vi "PID Initializer.vi"(8 "error in":errorcluster, 10 "PIDF":cluster{"P":dbl, "I":dbl, "D":dbl, "F":dbl} {"F" format="%#_13g"; "D" format="%#_13g"; "I" format="%#_13g"; "P" format="%#_13g"}, 11 "Can IDs":T7) -> (0 "error out":errorcluster, 3 "Motors":T6)   [LabVIEW 2020]
uses:
  <vilib>/Rock Robotics/WPI/MotorControl/WPI_MotorControlDeviceRef.ctl
  <vilib>/Rock Robotics/WPI/MotorControl/WPI_MotorControlType.ctl
  <vilib>/Rock Robotics/SystemInterfaces/DIO/FPGA_DIOPWMChannel.ctl
  <vilib>/Rock Robotics/WPI/PWM/WPI_PWMDeadband.ctl
  <vilib>/Rock Robotics/SystemInterfaces/DIO/FPGA_DIOChannel.ctl
  <vilib>/Rock Robotics/WPI/ThirdParty/Phoenix-LabVIEW/Motor Controller/Controls/CTRE_Phoenix_MotorControl_NeutralMode.ctl
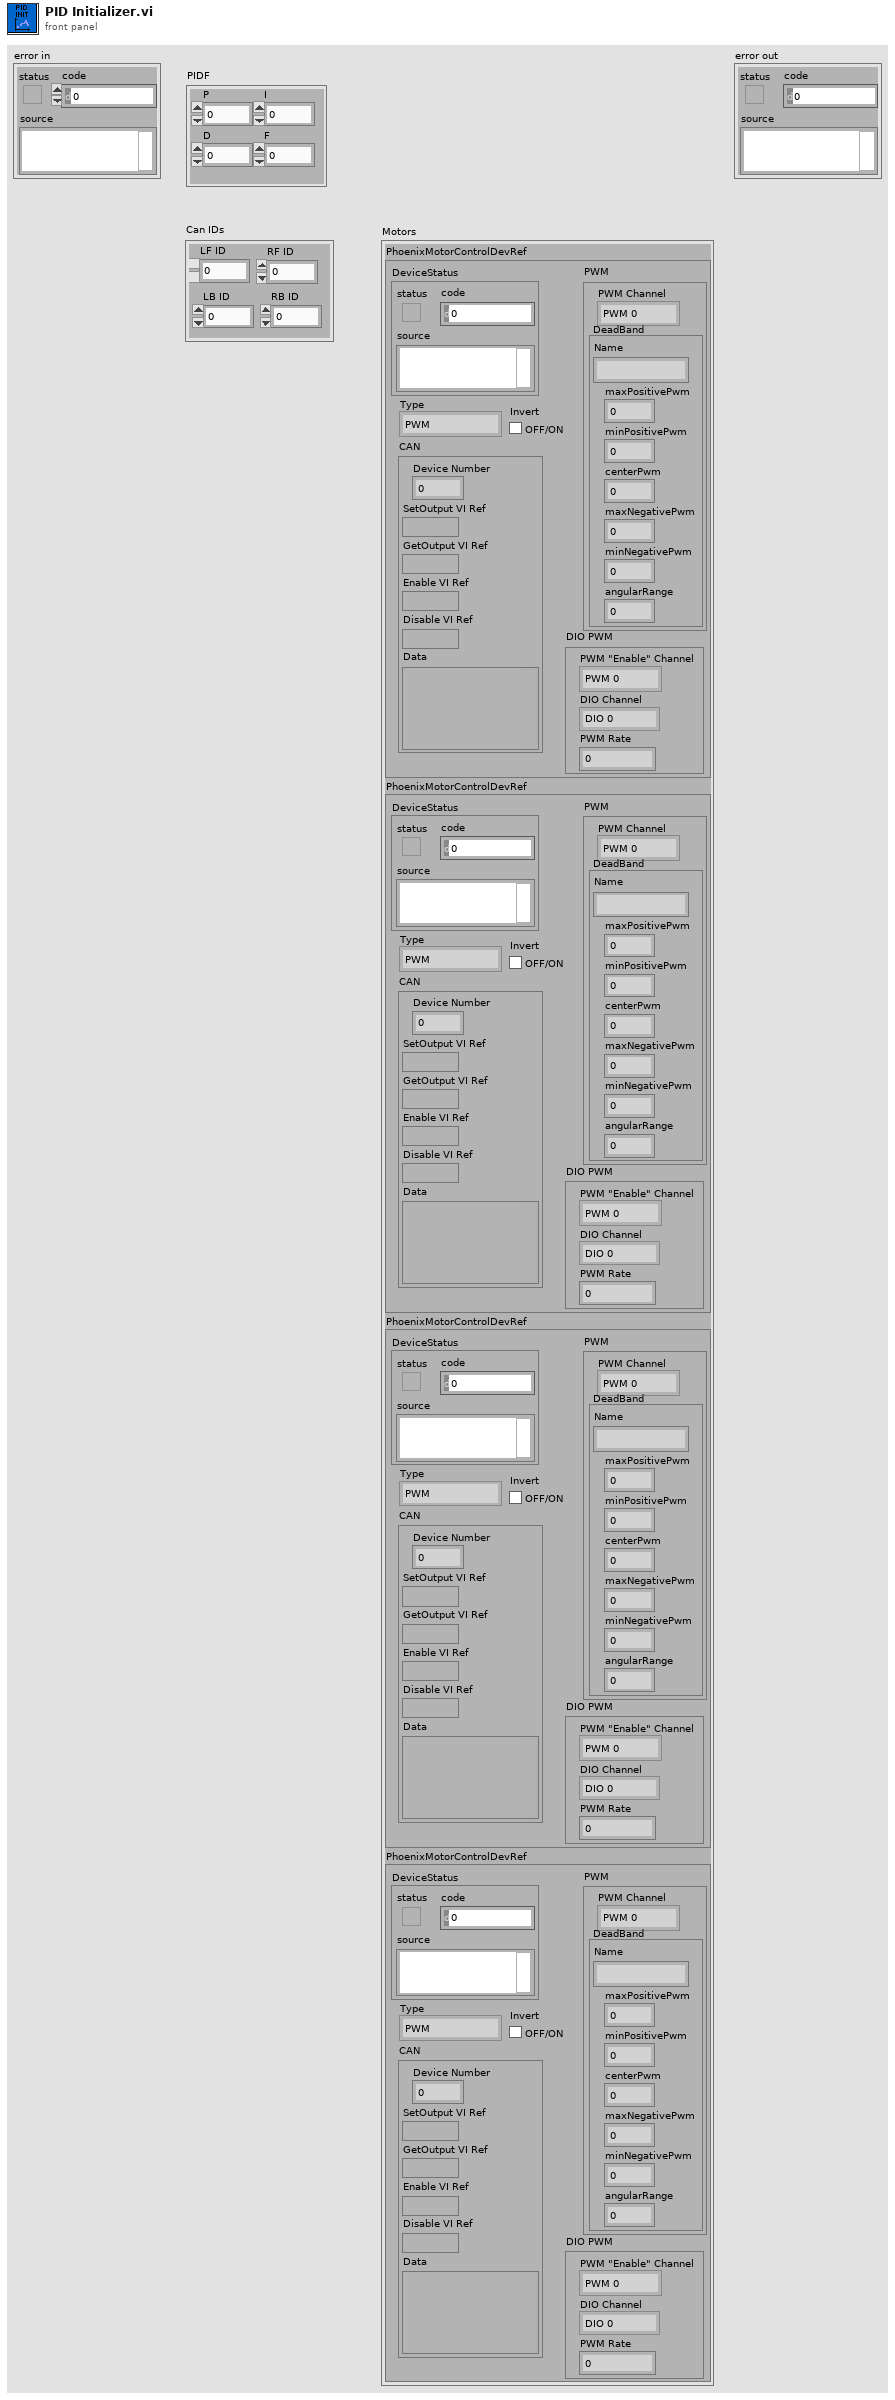
[diagram p1: front panel]
types:
  T1 = typedef "WPI_MotorControlDeviceRef.ctl" = cluster{"DeviceStatus":errorcluster, "Type":T2, "PWM":cluster{"PWM Channel":T3, "DeadBand":T4}, "CAN":cluster{"Device Number":u8, "SetOutput VI Ref":variant, "GetOutput VI Ref":variant, "Enable VI Ref":variant, "Disable VI Ref":variant, "Data":variant}, "Invert":bool, "DIO PWM":cluster{"PWM \"Enable\" Channel":T3, "DIOChannel":T5, "PWM Rate":dbl}}
  T2 = typedef "WPI_MotorControlType.ctl" = enum16{"PWM", "CAN", "DIO PWM"}
  T3 = typedef "FPGA_DIOPWMChannel.ctl" = enum8{"PWM 0", "PWM 1", "PWM 2", "PWM 3", "PWM 4", "PWM 5", "PWM 6", "PWM 7", "PWM 8", "PWM 9", "PWM MXP 0", "PWM MXP 1", "PWM MXP 2", "PWM MXP 3", "PWM MXP 4", "PWM MXP 5", "PWM MXP 6", "PWM MXP 7", "PWM MXP 8", "PWM MXP 9", "Invalid"}
  T4 = typedef "WPI_PWMDeadband.ctl" = cluster{"Name":string, "maxPositivePwm":i32, "minPositivePwm":i32, "centerPwm":i32, "maxNegativePwm":i32, "minNegativePwm":i32, "angularRange":u16}
  T5 = typedef "FPGA_DIOChannel.ctl" = enum8{"DIO 0", "DIO 1", "DIO 2", "DIO 3", "DIO 4", "DIO 5", "DIO 6", "DIO 7", "DIO 8", "DIO 9", "DIO MXP 0", "DIO MXP 1", "DIO MXP 2", "DIO MXP 3", "DIO MXP 4", "DIO MXP 5", "DIO MXP 6", "DIO MXP 7", "DIO MXP 8", "DIO MXP 9", "DIO MXP 10", "DIO MXP 11", "DIO MXP 12", "DIO MXP 13", "DIO MXP 14", "DIO MXP 15", "SPI Port CS1", "SPI Port CS2", "SPI Port CS3", "SPI Port MISO", "SPI Port MOSI", "Invalid"}
  T6 = cluster{"PhoenixMotorControlDevRef":T1, "PhoenixMotorControlDevRef":T1, "PhoenixMotorControlDevRef":T1, "PhoenixMotorControlDevRef":T1}
  T7 = cluster{"LF ID":u8, "LB ID":u8, "RF ID":u8, "RB ID":u8}
  T8 = typedef "CTRE_Phoenix_MotorControl_NeutralMode.ctl" = enum8{"EEPROMSetting", "Override to Coast", "Override to Brake"}
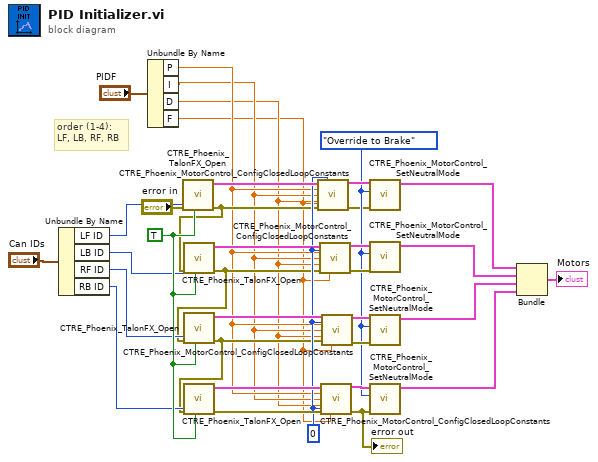
[diagram p0: block diagram]
diagram:
  w8 = CTRE_Phoenix_MotorControl_NeutralMode."Override to Brake" ("Motor Control Neutral Mode")
  w29 = 0 ("slotIdx")
  w30 = TRUE ("Invert")
  # "order (1-4):\nLF, LB, RF, RB"
  n1 = Unbundle By Name("Can IDs") -> ("LF ID"=w27:u8, "LB ID"=w26:u8, "RF ID"=w25:u8, "RB ID"=w24:u8)
  n2 = Unbundle By Name("PIDF") -> ("P"=w19:dbl, "I"=w18:dbl, "D"=w17:dbl, "F"=w16:dbl)
  n3 = call <vilib>:"CTRE_Phoenix_TalonFX_Open.vi"("Invert"=w30, "error in"="error in", "Device Number"=w27) -> ("error out"=w23:errorcluster, "PhoenixMotorControlDevRef"=w35:T1)  [unwired: 7 in]
  n4 = call <vilib>:"CTRE_Phoenix_TalonFX_Open.vi"("Invert"=w30, "error in"=w23, "Device Number"=w26) -> ("error out"=w22:errorcluster, "PhoenixMotorControlDevRef"=w34:T1)  [unwired: 7 in]
  n5 = call <vilib>:"CTRE_Phoenix_TalonFX_Open.vi"("Invert"=w30, "error in"=w22, "Device Number"=w25) -> ("error out"=w21:errorcluster, "PhoenixMotorControlDevRef"=w33:T1)  [unwired: 7 in]
  n6 = call <vilib>:"CTRE_Phoenix_TalonFX_Open.vi"("Invert"=w30, "error in"=w21, "Device Number"=w24) -> ("error out"=w31:errorcluster, "PhoenixMotorControlDevRef"=w32:T1)  [unwired: 7 in]
  n7 = call <vilib>:"CTRE_Phoenix_MotorControl_ConfigClosedLoopConstants.vi"("PhoenixMotorControlDevRef"=w35, "slotIdx"=w29, "P"=w19, "I"=w18, "D"=w17, "error in (no error)"=w23, "F"=w16) -> ("PhoenixMotorControlDevRef"=w9:T1, "error out"=w3:errorcluster)  [unwired: 7 in]
  n8 = call <vilib>:"CTRE_Phoenix_MotorControl_ConfigClosedLoopConstants.vi"("PhoenixMotorControlDevRef"=w34, "slotIdx"=w29, "P"=w19, "I"=w18, "D"=w17, "error in (no error)"=w22, "F"=w16) -> ("PhoenixMotorControlDevRef"=w13:T1, "error out"=w14:errorcluster)  [unwired: 7 in]
  n9 = call <vilib>:"CTRE_Phoenix_MotorControl_ConfigClosedLoopConstants.vi"("PhoenixMotorControlDevRef"=w32, "slotIdx"=w29, "P"=w19, "I"=w18, "D"=w17, "error in (no error)"=w31, "F"=w16) -> ("PhoenixMotorControlDevRef"=w10:T1, "error out"=w2:errorcluster)  [unwired: 7 in]
  "error out" <- w2
  n10 = call <vilib>:"CTRE_Phoenix_MotorControl_ConfigClosedLoopConstants.vi"("PhoenixMotorControlDevRef"=w33, "slotIdx"=w29, "P"=w19, "I"=w18, "D"=w17, "error in (no error)"=w21, "F"=w16) -> ("PhoenixMotorControlDevRef"=w11:T1, "error out"=w12:errorcluster)  [unwired: 7 in]
  n11 = call <vilib>:"CTRE_Phoenix_MotorControl_SetNeutralMode.vi"("error in (no error)"=w3, "Motor Control Neutral Mode"=w8, "PhoenixMotorControlDevRef"=w9) -> ("PhoenixMotorControlDevRef"=w7:T1)  [unwired: 7 in, 1 out]
  n12 = call <vilib>:"CTRE_Phoenix_MotorControl_SetNeutralMode.vi"("error in (no error)"=w14, "Motor Control Neutral Mode"=w8, "PhoenixMotorControlDevRef"=w13) -> ("PhoenixMotorControlDevRef"=w6:T1)  [unwired: 7 in, 1 out]
  n13 = call <vilib>:"CTRE_Phoenix_MotorControl_SetNeutralMode.vi"("error in (no error)"=w12, "Motor Control Neutral Mode"=w8, "PhoenixMotorControlDevRef"=w11) -> ("PhoenixMotorControlDevRef"=w5:T1)  [unwired: 7 in, 1 out]
  n14 = call <vilib>:"CTRE_Phoenix_MotorControl_SetNeutralMode.vi"("error in (no error)"=w2, "Motor Control Neutral Mode"=w8, "PhoenixMotorControlDevRef"=w10) -> ("PhoenixMotorControlDevRef"=w4:T1)  [unwired: 7 in, 1 out]
  n15 = Bundle("PhoenixMotorControlDevRef"=w7, "PhoenixMotorControlDevRef"=w6, "PhoenixMotorControlDevRef"=w5, "PhoenixMotorControlDevRef"=w4) -> (→"Motors":T6)  [unwired: 1 in]
